vi "Stream Wait for Input (Analog).vi"(4 "Reference Value (0)":dbl min=0.0 step=0.0001 format="%#.1g", 6 "Condition (0: ==)":u16(ring) items=["==", "<>", "<", ">", "<=", ">="], 7 "Pin Number (1)":u8=1, 8 "error in (no error)":errorcluster, 9 "Device Number":string, 10 "Stream Number (1)":u8=1, 11 "VISA resource name":refnum<visa-resource-name>) -> (0 "error out":errorcluster, 3 "VISA resource name out":refnum<visa-resource-name>)   [LabVIEW 2015, in "Zaber A Series.lvlib"]
doc: "Causes stream processing to pause until an analog input condition has been met. The controller will monitor its input pins until the condition is satisfied. The reference input value is in volts.\n\nThis VI does not check in advance for error conditions such as streams not being supported.\n\nThis VI requires that the Initialize VI has been called with the same serial port and that the specified stream buffer has already been opened."
uses:
  Zaber A Series.lvlib
  Private/All Commands.ctl
panel:
  out "Hidden indicator":u16(ring) items=["==", "<>", "<", ">", "<=", ">="]
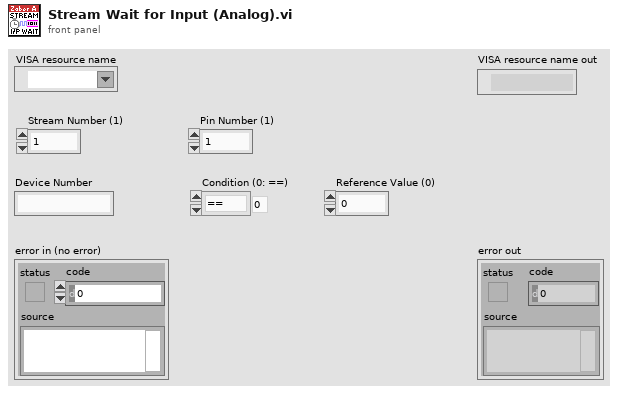
[diagram p1: front panel]
types:
  T1 = typedef "Zaber A Series.lvlib/All Commands.ctl" = string
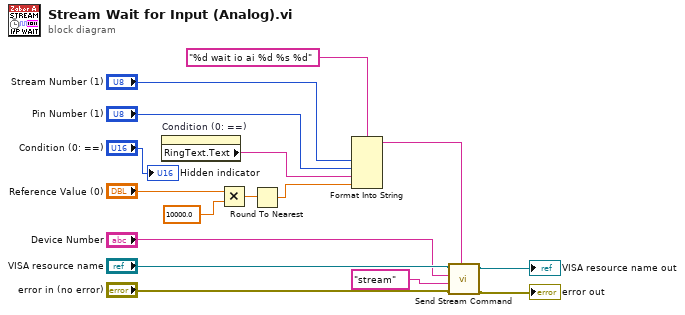
[diagram p0: block diagram]
diagram:
  n1 = property on="Condition (0: ==)" class="Ring (strict)"() -> ("RingText.Text"=w5:string)  [unwired: 2 in, 2 out]
  n2 = Multiply(x="Reference Value (0)", y=10000.0) -> (x*y=w9:dbl)
  n3 = Round To Nearest(number=w9) -> (nearest integer value=w4:dbl)
  n4 = Format Into String(format string="%d wait io ai %d %s %d", "Stream Number (1)", "Pin Number (1)", w5, w4) -> (resulting string=w3:string)  [unwired: 2 in, 1 out]
  n5 = call "Send Stream Command.vi"("Data"=w3, "error in (no error)"="error in (no error)", "Command"=T1 "stream" ("Complete Command List"), "Device Number"="Device Number", "VISA resource name"="VISA resource name") -> ("error out"=→"error out":errorcluster, "VISA resource name out"=→"VISA resource name out":refnum<visa-resource-name>)  [unwired: 5 in]
  "Hidden indicator" <- "Condition (0: ==)"
